vi "Open.vi"(8 "error in (no error)":errorcluster, 9 "Timeout (3s)":i32=3, 10 "Baud (115200)":i32=115200, 11 "Serial Port":string) -> (0 "error out":errorcluster, 2 "Success?":bool, 3 "Handle out":i32)   [LabVIEW 2013, in "Thorlabs_MC2000B.lvlib"]
uses:
  <instrlib>/Thorlabs_MC2000B/Thorlabs_MC2000B.lvlib
  <instrlib>/Thorlabs_MC2000B/Library/MC2000CommandLibWin64.dll
  <instrlib>/Thorlabs_MC2000B/Library/MC2000CommandLibWin32.dll
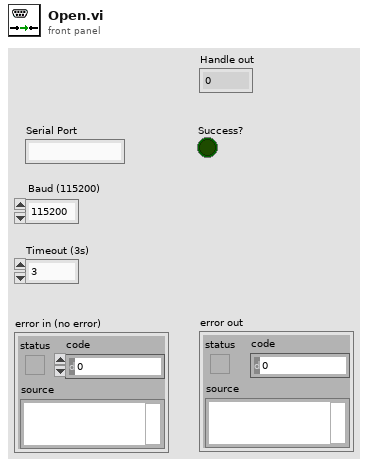
[diagram p1: front panel]
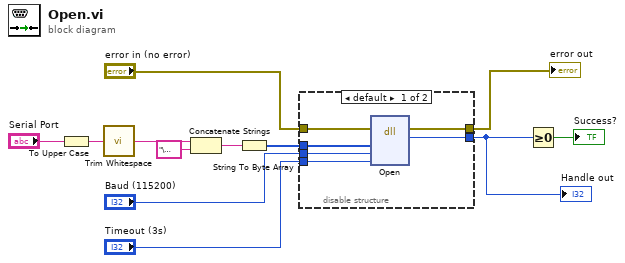
[diagram p0: block diagram]
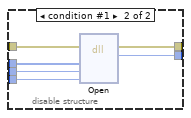
[diagram p2: hidden frame]
diagram:
  n1 = To Upper Case(1:"Serial Port") -> (0:w6:string)
  n2 = call <vilib>:"Trim Whitespace.vi"("string"=w6) -> ("trimmed string"=w5:string)  [unwired: 1 in]
  n3 = Concatenate Strings(w5, "\u0000" ("string")) -> (w2:string)
  n4 = String To Byte Array(string=w2) -> (unsigned byte array=w3:u8[])
  n5 = disable-structure shown="default" {
    disable-tunnel: "Baud (115200)" -> [w18 w24]
    disable-tunnel: "Timeout (3s)" -> [w17 w23]
    disable-tunnel: "error in (no error)" -> [w16 w22]
    disable-tunnel: [w15 w21] -> w7
    disable-tunnel: w3 -> [w14 w20]
    disable-tunnel: [w13 w19] -> w4
    frame condition #0 (active) {
      n6 = dll-call lib="C:/Program Files (x86)/National Instruments/LabVIEW 2013/instr.lib/Thorlabs_MC2000B/Library/MC2000CommandLibWin32.dll" fn="Open"(error in=w16, "nPort"=w14, "nBaud"=w18, "Time"=w17) -> (error out=w15:errorcluster, "return type"=w13:i32)  [unwired: 5 in, 1 out]
    }
    frame condition #1 {
      n7 = dll-call lib="D:/Program Files/National Instruments/LabVIEW 2011/instr.lib/Thorlabs_MC2000B/Library/MC2000CommandLibWin64.dll" fn="Open"(error in=w22, "nPort"=w20, "nBaud"=w24, "Time"=w23) -> (error out=w21:errorcluster, "return type"=w19:i32)  [unwired: 5 in, 1 out]
    }
  }
  "error out" <- w7
  "Handle out" <- w4
  n8 = Greater Or Equal To 0?(x=w4) -> (x >= 0?=→"Success?":bool)
